vi "Orca Flash Sort Filenames.vi"(7 "Requested File Path":path) -> (8 "Resulting File Path":path)   [LabVIEW 2025]
uses:
  kernel32.dll
  shell32.dll
panel:
  out "ReName Success?":bool
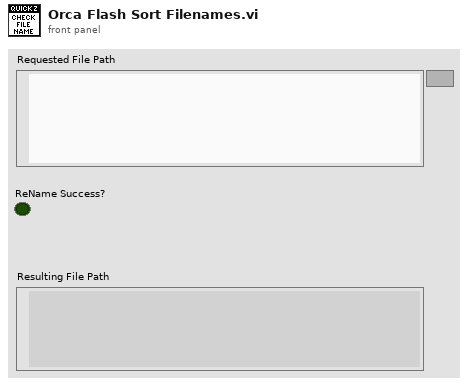
[diagram p1: front panel]
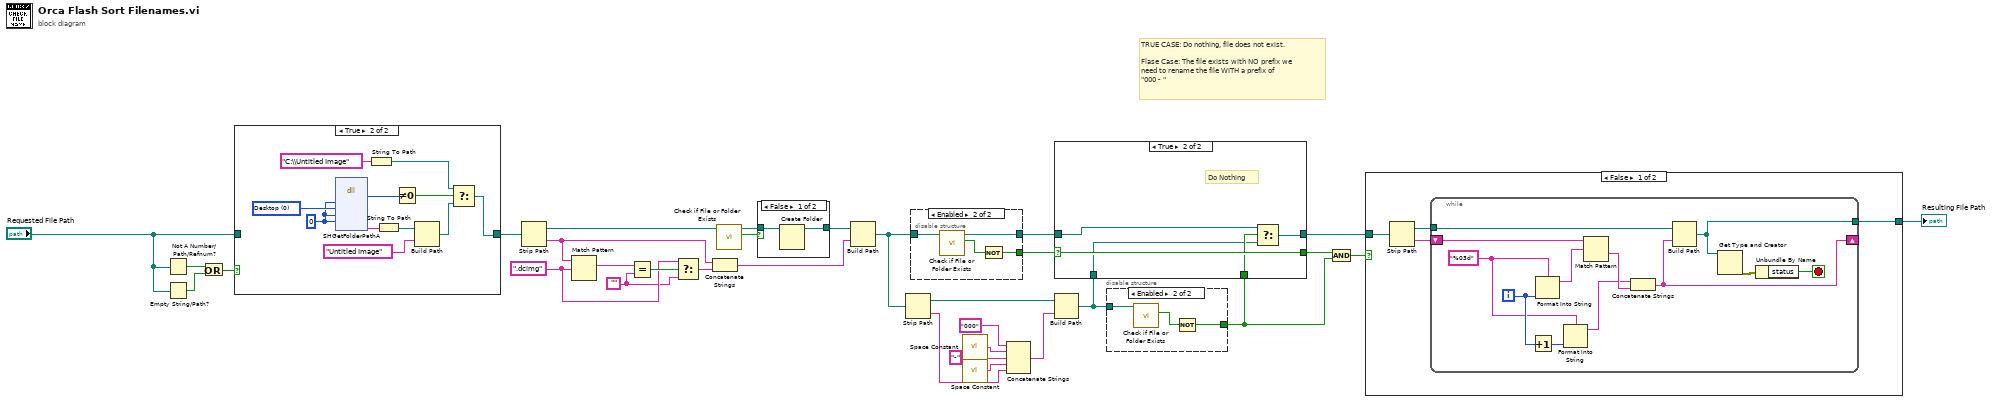
[diagram p0: block diagram]
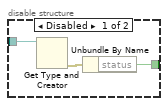
[diagram p2: hidden frame]
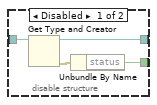
[diagram p3: hidden frame]
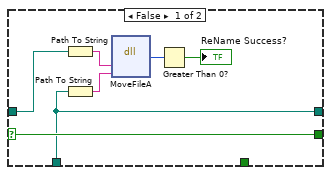
[diagram p6: hidden frame]
diagram:
  w12 = ""
  w13 = ".dcimg" ("regular expression")
  # "TRUE CASE: Do nothing, file does not exist.\n\nFlase Case: The file exists with NO prefix we\nneed to rename the file WITH a prefix of\n\"000 - \""
  n1 = Not A Number/Path/Refnum?(number/path/refnum="Requested File Path") -> (NaN/Path/Refnum?=w9:bool)
  n2 = Empty String/Path?(string/path="Requested File Path") -> (empty?=w1:bool)
  n3 = Or(x=w9, y=w1) -> (x .or. y?=w8:bool)
  n4 = case shown="True" w8 {
    tunnel: "Requested File Path" -> [w33 _]
    tunnel: [w33 w34] -> w7
    frame False {
    }
    frame True {
      w44 = 0 items=["Desktop"=0, "Personal Documents"=5, "AppData"=26, "Local AppData"=28, "Common AppData"=35, "Program Files"=38, "Program Files Common"=43, "Common Documents"=46] ("Requested Path")
      w43 = 0 ("HWND")
      n5 = dll-call lib="shell32.dll" fn="SHGetFolderPathA"("HWND"=w43, "nFolder"=w44, "hToken"=w43, "dwFlags"=w43) -> ("Succeeded"=w39:i32, "pszPath"=w42:string)  [unwired: 8 in, 2 out]
      n6 = String To Path(string="C:\\Untitled Image" ("regular expression")) -> (path=w36:path)
      n7 = String To Path(string=w42) -> (path=w41:path)
      n8 = Not Equal To 0?(x=w39) -> (x != 0?=w37:bool)
      n9 = Build Path(base path=w41, name or relative path="Untitled Image" ("regular expression")) -> (appended path=w35:path)
      n10 = Select(t=w36, s=w37, f=w35) -> (s? t:f=w34:path)
    }
  }
  n11 = Strip Path(path=w7) -> (stripped path=w4:path, name=w14:string)
  n12 = Match Pattern(string=w14, regular expression=w13) -> (match substring=w17:string)  [unwired: 1 in, 3 out]
  n13 = Equal?(x=w17, y=w12) -> (x = y?=w16:bool)
  n14 = Select(t=w13, s=w16, f=w12) -> (s? t:f=w15:string)
  n15 = Concatenate Strings(w14, w15) -> (w10:string)
  n16 = call <vilib>:"Check if File or Folder Exists.vi"("path"=w4) -> ("file or folder exists?"=w6:bool, "dup path"=w5:path)  [unwired: 8 in, 1 out]
  n17 = case shown="False" w6 {
    tunnel: [w45 w47] -> w3
    tunnel: w5 -> [w46 w47]
    frame False {
      n18 = Create Folder(path (use dialog)=w46) -> (created path=w45:path)  [unwired: 2 in, 2 out]
    }
    frame True {
    }
  }
  n19 = Build Path(base path=w3, name or relative path=w10) -> (appended path=w11:path)
  n20 = Strip Path(path=w11) -> (stripped path=w29:path, name=w25:string)
  n21 = disable-structure shown="Enabled" {
    disable-tunnel: [w50 w52] -> w23
    disable-tunnel: [w49 w54] -> w21
    disable-tunnel: w11 -> [w48 w55]
    frame Disabled {
      n22 = Get Type and Creator(7:w48) -> (0:w51:errorcluster, 3:w49:path)  [unwired: 1 in, 2 out]
      n23 = Unbundle By Name(w51) -> ("status"=w50:bool)
    }
    frame Enabled {
      n24 = call <vilib>:"Check if File or Folder Exists.vi"("path"=w55) -> ("file or folder exists?"=w53:bool, "dup path"=w54:path)  [unwired: 8 in, 1 out]
      n25 = Not(x=w53) -> (.not. x?=w52:bool)
    }
  }
  n26 = call <vilib>:"Space Constant.vi"() -> ("String"=w31:string)
  n27 = call <vilib>:"Space Constant.vi"() -> ("String"=w27:string)
  n28 = Concatenate Strings("000", w31, "-", w27, w25) -> (w28:string)
  n29 = Build Path(base path=w29, name or relative path=w28) -> (appended path=w19:path)
  n30 = disable-structure shown="Enabled" {
    disable-tunnel: w19 -> [w57 w61]
    disable-tunnel: [w56 w59] -> w18
    frame Disabled {
      n31 = Get Type and Creator(7:w57) -> (0:w58:errorcluster)  [unwired: 1 in, 3 out]
      n32 = Unbundle By Name(w58) -> ("status"=w56:bool)
    }
    frame Enabled {
      n33 = call <vilib>:"Check if File or Folder Exists.vi"("path"=w61) -> ("file or folder exists?"=w60:bool)  [unwired: 8 in, 2 out]
      n34 = Not(x=w60) -> (.not. x?=w59:bool)
    }
  }
  n35 = case shown="True" w23 {
    selector: w23 -> [w68 w73]
    tunnel: [w68 w73] -> w22
    tunnel: w21 -> [w63 w71]
    tunnel: [w62 w70] -> w20
    tunnel: w19 -> [w62 w69]
    tunnel: w18 -> [_ w72]
    frame False {
      n36 = Path To String(path=w63) -> (string=w65:string)
      n37 = Path To String(path=w62) -> (string=w64:string)
      n38 = dll-call lib="kernel32.dll" fn="MoveFileA"(w65, w64) -> ("return type"=w66:i32)  [unwired: 5 in, 2 out]
      n39 = Greater Than 0?(x=w66) -> (x > 0?=→"ReName Success?":bool)
    }
    frame True {
      # "Do Nothing"
      n40 = Select(t=w71, s=w72, f=w69) -> (s? t:f=w70:path)
    }
  }
  n41 = And(x=w22, y=w18) -> (x .and. y?=w24:bool)
  n42 = case shown="False" w24 {
    tunnel: w20 -> [w77 w90]
    tunnel: [w74 w90] -> w32
    frame False {
      n43 = Strip Path(path=w77) -> (stripped path=w76:path, name=w75:string)
      n44 = while {
        tunnel: w76 -> [w88]
        tunnel: [w85] -> w74
        shift-right: [w78] -> _
        shift-left: w75 -> [w89]
        i -> [w82]
        stop <- w83 stop-if-true
        w80 = "%03d" ("format string")
        n45 = Increment(x=w82) -> (x+1=w81:i32)
        n46 = Format Into String(format string=w80, w82) -> (resulting string=w87:string)  [unwired: 2 in, 1 out]
        n47 = Format Into String(format string=w80, w81) -> (resulting string=w79:string)  [unwired: 2 in, 1 out]
        n48 = Match Pattern(string=w89, regular expression=w87) -> (after substring=w86:string)  [unwired: 1 in, 3 out]
        n49 = Concatenate Strings(w79, w86) -> (w78:string)
        n50 = Build Path(base path=w88, name or relative path=w78) -> (appended path=w85:path)
        n51 = Get Type and Creator(7:w85) -> (0:w84:errorcluster)  [unwired: 1 in, 3 out]
        n52 = Unbundle By Name(w84) -> ("status"=w83:bool)
      }
    }
    frame True {
      # "File does NOT exist - Do NOTHING"
    }
  }
  "Resulting File Path" <- w32
